vi "Camera 0 Control AE.vi"(1 "Camera Control Input":T2 {"Frame Rate (fps)" scale=6.1..17.45; "Exposure Time (ms)" scale=0.06..1.0; "Pixel Clock (MHz)" scale=5.0..43.0}, 2 "Action":T1) -> (0 "Camera Control Output":T2 {"Frame Rate (fps)" scale=6.1..17.45; "Exposure Time (ms)" scale=0.06..1.0; "Pixel Clock (MHz)" scale=5.0..43.0})   [LabVIEW 2014]
uses:
  Focus Lock/Controls/Camera Control.ctl
  Focus Lock/Controls/Standard Action for Focus Lock.ctl
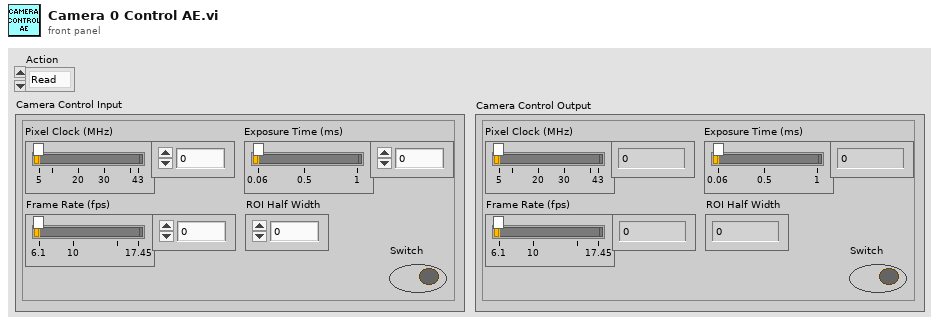
[diagram p1: front panel]
types:
  T1 = typedef "Standard Action for Focus Lock.ctl" = enum16{"Read", "Write"}
  T2 = typedef "Camera Control.ctl" = cluster{"Pixel Clock (MHz)":i32, "Exposure Time (ms)":dbl, "Frame Rate (fps)":dbl, "ROI Half Width":i32, "Switch":bool}
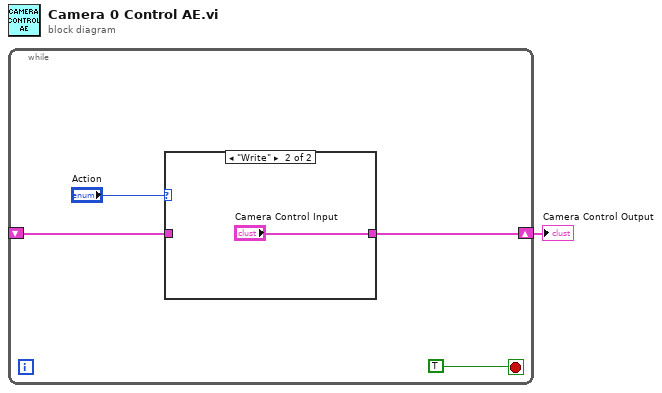
[diagram p0: block diagram]
diagram:
  n1 = while {
    shift-right: [w5] -> w1
    shift-left: _ -> [w4]
    stop <- TRUE stop-if-true
    n2 = case shown="\"Write\"" "Action" {
      tunnel: [w6 "Camera Control Input"] -> w5
      tunnel: w4 -> [w6 _]
      frame "Read", Default {
      }
      frame "Write" {
      }
    }
  }
  "Camera Control Output" <- w1
